vi "cycle sort file.vi"(8 "error in":errorcluster, 11 "file path (dialog if empty)":path) -> (0 "error out":errorcluster, 3 "cycle results cluster":T1, 4 "new file path (Not A Path if cancelled)":path)   [LabVIEW 2016]
doc: "takes the cycle information and sorts it into 3 arrays. A text array, a header array for the cycle information and a double array with the actual cycle information in it"
uses:
  controls/cycle results control.ctl
  <vilib>/Utility/file.llb/Read From Spreadsheet File (string).vi
panel:
  out "first row":string[](array[string])
  out "all rows":string[][](array[string])
  out "size(s)":i32[](array[numeric])
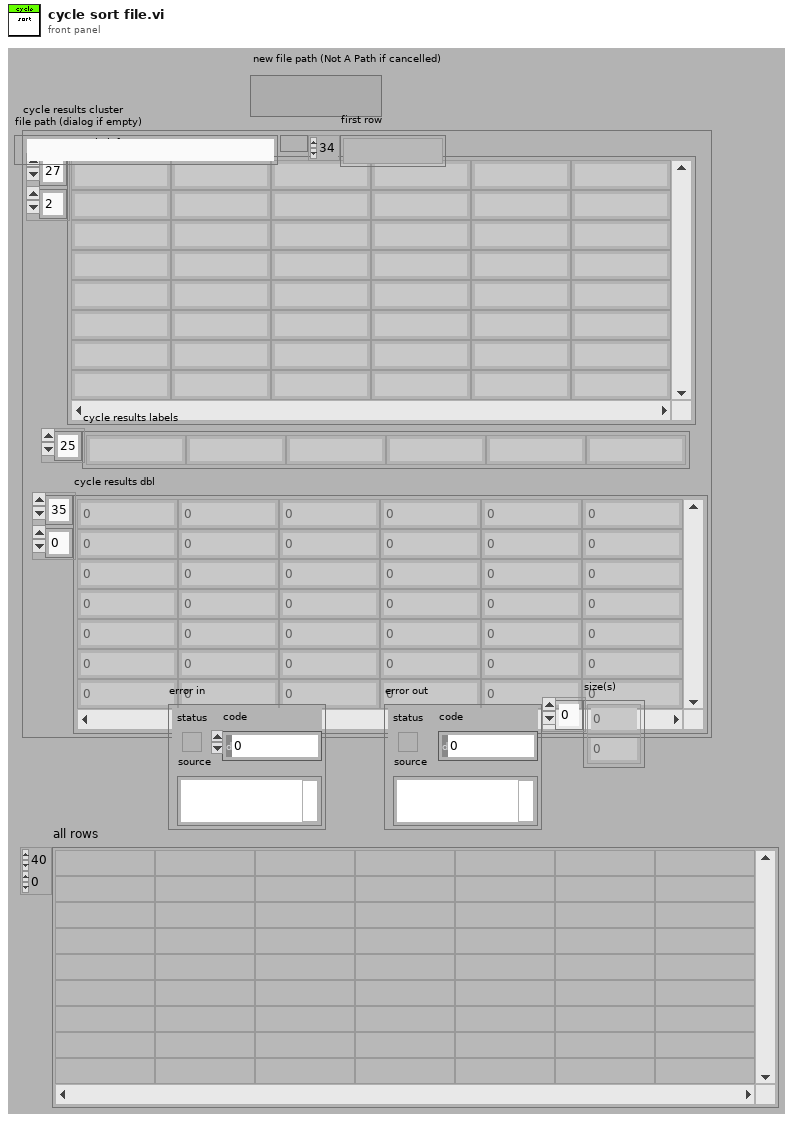
[diagram p1: front panel]
types:
  T1 = typedef "cycle results control.ctl" = cluster{"sample info":string[][], "cycle results labels":string[], "cycle results dbl":dbl[][]}
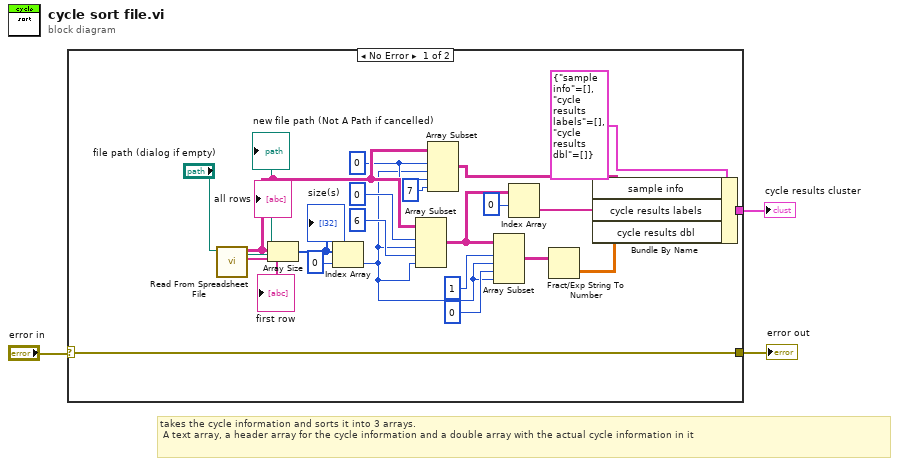
[diagram p0: block diagram]
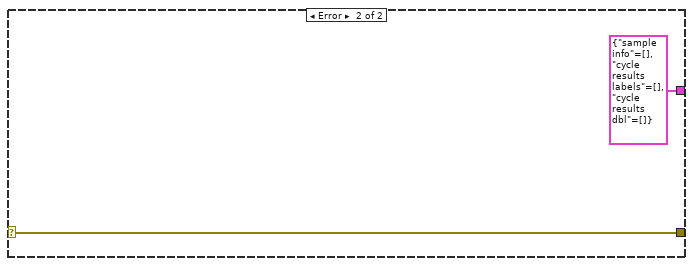
[diagram p2: hidden frame]
diagram:
  # "takes the cycle information and sorts it into 3 arrays. \n A text array, a header array for the cycle information and a double array with the actual cycle information in it"
  n1 = case shown="No Error" "error in" {
    selector: "error in" -> [w9 w27]
    tunnel: [w25 T1 {"sample info"=[], "cycle results labels"=[], "cycle results dbl"=[]} ("cycle results cluster")] -> w3
    tunnel: [w9 w27] -> w1
    frame No Error {
      w13 = 0 ("index")
      n2 = call-poly <vilib>:"Read From Spreadsheet File.vi"("file path (dialog if empty)"="file path (dialog if empty)") -> ("first row"=→"first row":string[], "all rows"=w14:string[][], "new file path (Not A Path if cancelled)"=→"new file path (Not A Path if cancelled)":path)  [unwired: 6 in, 2 out]
      "all rows" <- w14
      n3 = Array Size(array=w14) -> (size(s)=w11:i32[])
      "size(s)" <- w11
      n4 = Index Array(array=w11, index=0) -> (element=w4:i32)
      n5 = Array Subset(array=w14, index (row)=0 ("length"), length (row)=w4, index (col)=6 ("index"), length (col)=w4) -> (w21:string[][])
      n6 = Array Subset(array=w14, index (row)=w13, length (row)=w4, index (col)=w13, length (col)=7 ("length")) -> (w23:string[][])
      n7 = Array Subset(array=w21, index (row)=1 ("index"), length (row)=w4, index (col)=0 ("index"), length (col)=w4) -> (w8:string[][])
      n8 = Index Array(array=w21, index (row)=0) -> (element=w24:string[])  [unwired: 1 in]
      n9 = Fract/Exp String To Number(string=w8) -> (number=w7:dbl[][])  [unwired: 3 in, 1 out]
      n10 = Bundle By Name(cluster=T1 {"sample info"=[], "cycle results labels"=[], "cycle results dbl"=[]} ("cycle results cluster"), "sample info"=w23, "cycle results labels"=w24, "cycle results dbl"=w7) -> (w25:T1)
    }
    frame Error {
    }
  }
  "cycle results cluster" <- w3
  "error out" <- w1
